vi "提取滴速信息.vi"(1 "剩余药量":dbl, 2 "Y均值变化数组":dbl[](array[numeric])) -> (0 "滴速（滴/秒）":dbl)   [LabVIEW 2017]
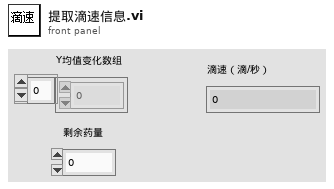
[diagram p1: front panel]
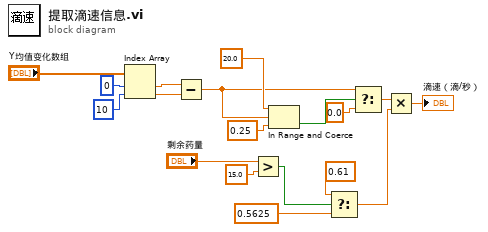
[diagram p0: block diagram]
diagram:
  n1 = Index Array(array="Y均值变化数组", index #1=0 ("索引"), index #2=10 ("索引")) -> (element #1=w8:dbl, element #2=w7:dbl)
  n2 = Subtract(x=w8, y=w7) -> (x-y=w14:dbl)
  n3 = Greater?(x="剩余药量", y=15.0) -> (0:w4:bool)
  n4 = In Range and Coerce(upper limit=20.0, x=w14, lower limit=0.25) -> (In Range?=w15:bool)  [unwired: 1 out]
  n5 = Select(t=0.61 ("y"), s=w4, f=0.5625 ("y")) -> (s? t:f=w1:dbl)
  n6 = Select(t=w14, s=w15, f=0.0) -> (s? t:f=w12:dbl)
  n7 = Multiply(x=w12, y=w1) -> (x*y=→"滴速（滴/秒）":dbl)
